vi "Projectx.vi"() -> ()   [LabVIEW 2020]
uses:
  <vilib>/event_ctls.llb/eventsource.ctl
panel:
  out "output cluster":cluster{"Source":T1, "BoolText.Text":string} {"Source" items=["LabVIEW UI"=0, "ActiveX"=1, "User Event"=25]}
  out "Output":string
  in  "Current Time":bool
  in  "Clear":bool
  in  "Stop":bool
  out "Loop Number":i32
  in  "Increment":bool
  # "LOOP FUNCTIONS"
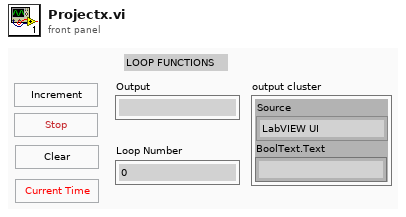
[diagram p1: front panel]
types:
  T1 = typedef "eventsource.ctl" = u32
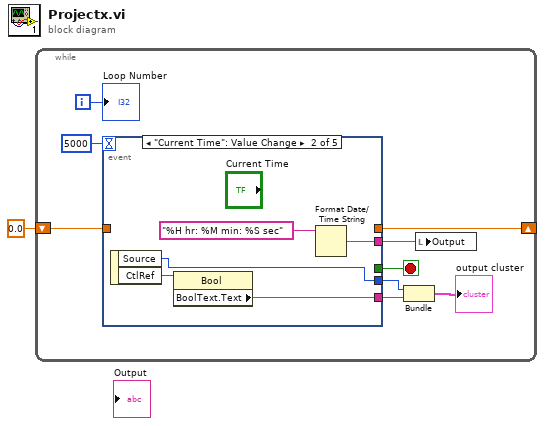
[diagram p0: block diagram]
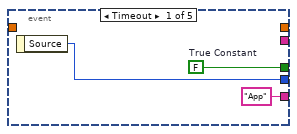
[diagram p2: hidden frame]
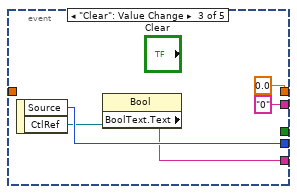
[diagram p3: hidden frame]
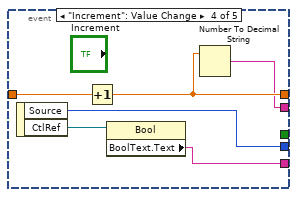
[diagram p4: hidden frame]
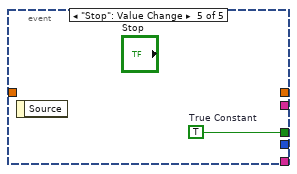
[diagram p5: hidden frame]
diagram:
  n1 = while {
    shift-right: [w9] -> _
    shift-left: 0.0 -> [w10]
    i -> [w8]
    stop <- w7 stop-if-true
    n2 = event shown="[1] \"Current Time\": Value Change" {
      selector: _ -> [_ _ _ _ _]
      dyn-events: _ -> [_ _ _ _ _]
      timeout: 5000 -> [_ _ _ _ _]
      tunnel: [_ _ 0.0 w25 _] -> w9
      tunnel: w10 -> [_ _ _ w29 _]
      tunnel: [w13 _ _ _ w30] -> w7
      tunnel: [_ w17 "0" ("date/time string") w24 _] -> w5
      tunnel: [w12 w15 w23 w26 _] -> w4
      tunnel: ["App" ("BoolText.Text") w14 w21 w27 _] -> w3
      event Timeout {
        w13 = FALSE  # True Constant
        n3 = event-data() -> ("Source"=w12:T1)  [unwired: 1 in]
      }
      event "Current Time": Value Change {
        n4 = event-data() -> ("Source"=w15:T1, "CtlRef"=w16:refnum<vi>)  [unwired: 1 in]
        n5 = property class="Bool"(reference=w16) -> ("BoolText.Text"=w14:string)  [unwired: 1 in, 2 out]
        n6 = Format Date/Time String(time format string (%c)="%H hr: %M min: %S sec") -> (date/time string=w17:string)  [unwired: 2 in]
      }
      event "Clear": Value Change {
        n7 = event-data() -> ("Source"=w23:T1, "CtlRef"=w22:refnum<vi>)  [unwired: 1 in]
        n8 = property class="Bool"(reference=w22) -> ("BoolText.Text"=w21:string)  [unwired: 1 in, 2 out]
      }
      event "Increment": Value Change {
        n9 = event-data() -> ("Source"=w26:T1, "CtlRef"=w28:refnum<vi>)  [unwired: 1 in]
        n10 = Increment(x=w29) -> (x+1=w25:dbl)
        n11 = property class="Bool"(reference=w28) -> ("BoolText.Text"=w27:string)  [unwired: 1 in, 2 out]
        n12 = Number To Decimal String(number=w25) -> (decimal integer string=w24:string)  [unwired: 1 in]
      }
      event "Stop": Value Change {
        w30 = TRUE  # True Constant
        n13 = event-data() -> ()  [unwired: 1 in, 1 out]
      }
    }
    n14 = Bundle("Source"=w4, "BoolText.Text"=w3) -> (→"output cluster":cluster{"Source":T1, "BoolText.Text":string})  [unwired: 1 in]
    n15 = local write "Output"(w5) -> ()
    "Loop Number" <- w8
  }
